vi "Human Control.vi"() -> ()   [LabVIEW 2009]
uses:
  <vilib>/userDefined/High Color/nirio_resource_hc.ctl
  FPGA/FPGA Opperation Mode.ctl
  <vilib>/rvi/interface/nirviOpenFPGA/nirviOpenFPGA.xnode
  Athena Human Control Code.lvbitx
  <vilib>/FPGAPlugInAG/sbRIO-9642/nirviIntfOpen_sbRIO-9642.vi
  <vilib>/rvi/interface/nirviReadWriteControl/nirviReadWriteControl.xnode
  <vilib>/Utility/error.llb/Error Cluster From Error Code.vi
  <vilib>/rvi/errors/niLvFpgaAdjustHostInterfaceError.vi
  <vilib>/rvi/interface/common/niFpgaNodeNameForErrorReporting.ctl
  <vilib>/rvi/errors/niLvFpgaWhatHappensToTopLevelVI.ctl
  <vilib>/rvi/interface/nirviCloseFPGA/nirviCloseFPGA.xnode
  <vilib>/FPGAPlugInAG/sbRIO-9642/nirviIntfClose_sbRIO-9642.vi
  NiRioSrv.dll
panel:
  in  "Turn Right":bool
  in  "Turn Left":bool
  in  "Forward":bool
  in  "Steering Position Offset":i32
  in  "Steering Enable":bool
  in  "Drive Enable":bool
  in  "Stop":bool
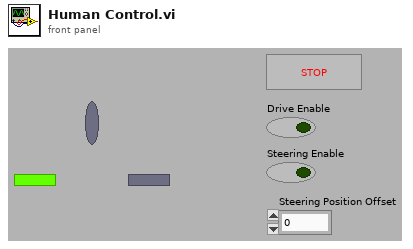
[diagram p1: front panel]
types:
  T1 = typedef "nirio_resource_hc.ctl" = tag
  T2 = typedef "FPGA Opperation Mode.ctl" = enum16{"Human Control"}
  T3 = typedef "niFpgaNodeNameForErrorReporting.ctl" = enum16{"Open FPGA VI Reference", "Read/Write Control", "Invoke Method: Abort", "Invoke Method: Acknowledge IRQ", "Invoke Method: Download", "Invoke Method: FIFO.Configure", "Invoke Method: FIFO.Read", "Invoke Method: FIFO.Start", "Invoke Method: FIFO.Stop", "Invoke Method: FIFO.Write", "Invoke Method: Reset", "Invoke Method: Run", "Invoke Method: Wait on IRQ", "Close FPGA VI Reference"}
  T4 = typedef "niLvFpgaWhatHappensToTopLevelVI.ctl" = enum16{"top level VI scripted behind XNode", "top level VI inlined behind XNode"}
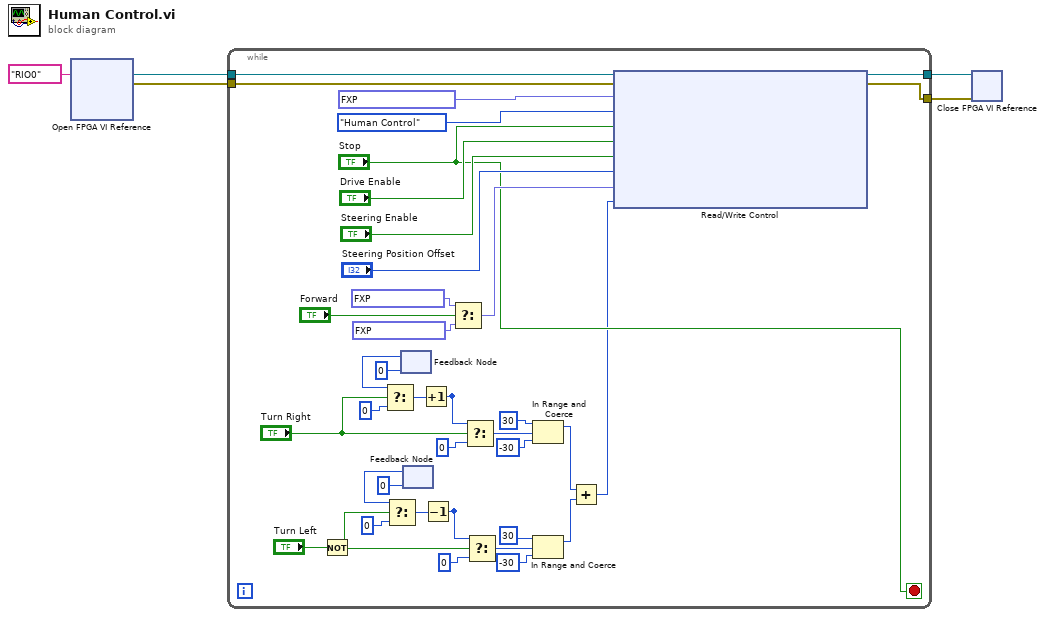
[diagram p0: block diagram]
diagram:
  n1 = xnode "Open FPGA VI Reference"("resource name"=T1 "RIO0") -> ("FPGA VI Reference Out"=w5:refnum<k20>, "error out"=w4:errorcluster)  [unwired: 1 in]
  n2 = while {
    tunnel: w5 -> [w43]
    tunnel: w4 -> [w42]
    tunnel: [w18] -> w3
    tunnel: [w17] -> w2
    stop <- "Stop" stop-if-true
    n3 = Not(x="Turn Left") -> (.not. x?=w13:bool)
    n4 = feedback #1(0 ("Steering Position Target")) -> (w32:i32)
    n5 = Select(t=w32, s="Turn Right", f=0 ("Steering Position Target")) -> (s? t:f=w29:i32)
    n6 = feedback #2(0 ("Steering Position Target")) -> (w21:i32)
    n7 = Select(t=w21, s=w13, f=0 ("Steering Position Target")) -> (s? t:f=w24:i32)
    n8 = Increment(x=w29) -> (x+1=w28:i32)
    n9 = Decrement(x=w24) -> (x-1=w19:i32)
    n10 = Select(t=fxp<+/-,18,8> 2.75 ("Drive Speed Current (1-3.5)"), s="Forward", f=fxp<+/-,18,8> 0.0 ("Drive Speed Current (1-3.5)")) -> (s? t:f=w33:fxp<+/-,18,8>)
    n11 = Select(t=w28, s="Turn Right", f=0 ("Steering Position Target")) -> (s? t:f=w12:i32)
    n12 = Select(t=w19, s=w13, f=0 ("Steering Position Target")) -> (s? t:f=w11:i32)
    n13 = In Range and Coerce(upper limit=30, x=w12, lower limit=-30) -> (coerced(x)=w9:i32)  [unwired: 1 out]
    n14 = In Range and Coerce(upper limit=30, x=w11, lower limit=-30) -> (coerced(x)=w10:i32)  [unwired: 1 out]
    n15 = Add(x=w9, y=w10) -> (x+y=w8:i32)
    n16 = xnode "Read/Write Control"("FPGA VI Reference In"=w43, "error in"=w42, "Steering Proportional Control Feedback Gain"=fxp<+/-,20,5> 0.100006103515625, "Enum"=FPGA_Opperation_Mode."Human Control", "Stop"="Stop", "Drive Enable"="Drive Enable", "Steering Enable"="Steering Enable", "Steering Position Offset"="Steering Position Offset", "Drive Speed Current (1-3.5)"=w33, "Steering Position Target"=w8) -> ("FPGA VI Reference Out"=w18:refnum<k20>, "error out"=w17:errorcluster)
  }
  n17 = xnode "Close FPGA VI Reference"("FPGA VI Reference In"=w3, "error in"=w2) -> ()  [unwired: 1 out]
